vi "USRP.vi"(6 "Active Antenna":string(combo)="RX1", 7 "Samples / Frame":i64=5000, 8 "Gain [dB]":dbl=20.0 format="%#.6p", 9 "Carrier\nFrequency [Hz]":dbl=90500000.0 format="%#.6p", 10 "IQ Sampling\nRate [S/sec]":dbl=200000.0 format="%#.6p", 11 "device name":refnum<k15>="192.168.10.2") -> (1 "error out":errorcluster, 2 "data":waveform(cdb), 3 "session handle out":refnum<k15>)   [LabVIEW 2015]
uses:
  <instrlib>/niUSRP/niUSRP Fetch Rx Data (CDB WDT).vi
panel:
  out "Gain [dB] (actual)":dbl=20.0 format="%#.6p"
  out "Carrier Frequency \n[Hz] (actual)":dbl=90499999.99533428 format="%#.6p"
  out "IQ Sampling\nRate [S/sec] (actual)":dbl=200000.0 format="%#.6p"
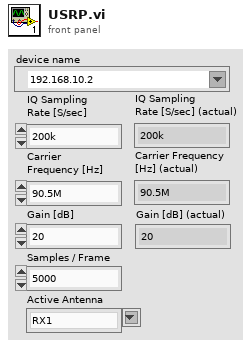
[diagram p1: front panel]
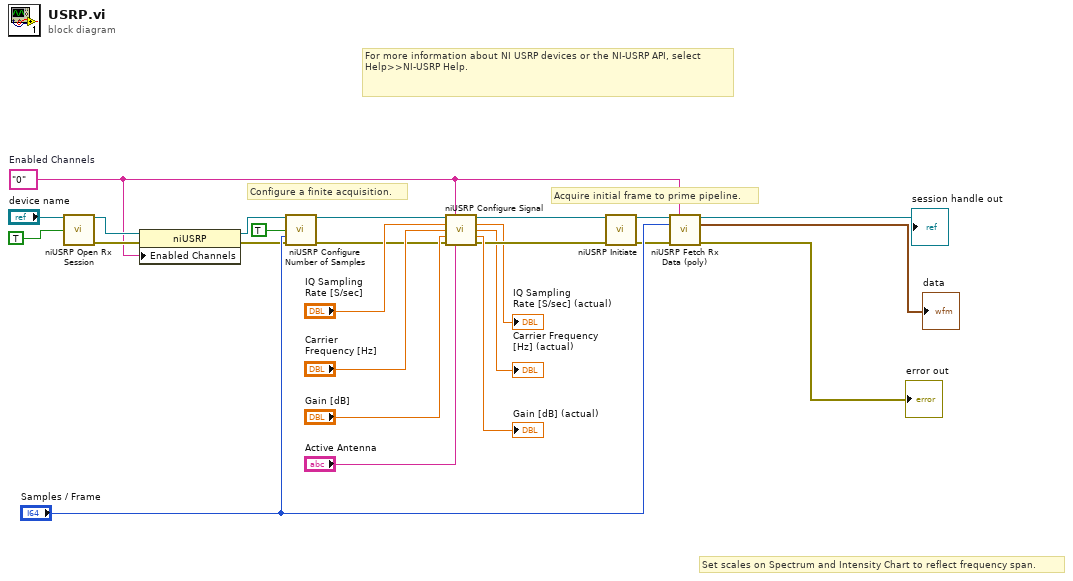
[diagram p0: block diagram]
diagram:
  w4 = "0"  # Enabled Channels
  # "For more information about NI USRP devices or the NI-USRP API, select Help>>NI-USRP Help."
  # "Acquire initial frame to prime pipeline."
  # "Configure a finite acquisition."
  # "Set scales on Spectrum and Intensity Chart to reflect frequency span."
  n1 = call <instrlib>:"niUSRP Open Rx Session.vi"("device names"="device name", "reset"=TRUE) -> ("session handle out"=w6:refnum<k15>, "error out"=w8:errorcluster)  [unwired: 12 in]
  n2 = property class="niUSRP"(reference=w6, error in=w8, "Enabled Channels"=w4) -> (reference out=w5:refnum<k15>, error out=w7:errorcluster)
  n3 = call <instrlib>:"niUSRP Configure Number of Samples.vi"("session handle"=w5, "number of samples is finite"=TRUE, "number of samples"="Samples / Frame", "error in (no error)"=w7) -> ("session handle out"=w19:refnum<k15>, "error out"=w18:errorcluster)  [unwired: 10 in]
  n4 = call <instrlib>:"niUSRP Configure Signal.vi"("session handle"=w19, "channel list"=w4, "IQ rate"="IQ Sampling\nRate [S/sec]", "carrier frequency"="Carrier\nFrequency [Hz]", "gain"="Gain [dB]", "error in (no error)"=w18, "active antenna"="Active Antenna") -> ("session handle out"=w16:refnum<k15>, "coerced IQ rate"=→"IQ Sampling\nRate [S/sec] (actual)":dbl, "coerced carrier frequency"=→"Carrier Frequency \n[Hz] (actual)":dbl, "coerced gain"=→"Gain [dB] (actual)":dbl, "error out"=w15:errorcluster)  [unwired: 4 in]
  n5 = call <instrlib>:"niUSRP Initiate.vi"("session handle"=w16, "error in (no error)"=w15) -> ("session handle out"=w12:refnum<k15>, "error out"=w13:errorcluster)  [unwired: 12 in]
  n6 = call-poly <instrlib>:"niUSRP Fetch Rx Data (poly).vi"("session handle"=w12, "channel list"=w4, "number of samples"="Samples / Frame", "error in (no error)"=w13) -> ("session handle out"=→"session handle out":refnum<k15>, "data"=→"data":waveform(cdb), "error out"=→"error out":errorcluster)  [unwired: 8 in, 1 out]
